vi "Strings and Values.vi"(8 "error in (no error)":errorcluster, 11 "NCDC Weather in":refnum<class "NCDC Weather.lvclass">) -> (0 "error out":errorcluster, 2 "Strings And Values []":T3, 3 "NCDC Weather out":refnum<class "NCDC Weather.lvclass">)   [LabVIEW 2020, in "NCDC Weather.lvclass"]
uses:
  NCDC Weather.lvclass
  <vilib>/Utility/miscctls.llb/LVComboBoxStrsAndValuesArrayTypeDef.ctl
  Location Result JSON.ctl
  Locations Results JSON.ctl
  NCDC Weather.lvclass/NCDC Weather.ctl
  <vilib>/httpClient/LabVIEWHTTPClient.lvlib
panel:
  out "Response (debug)":T1
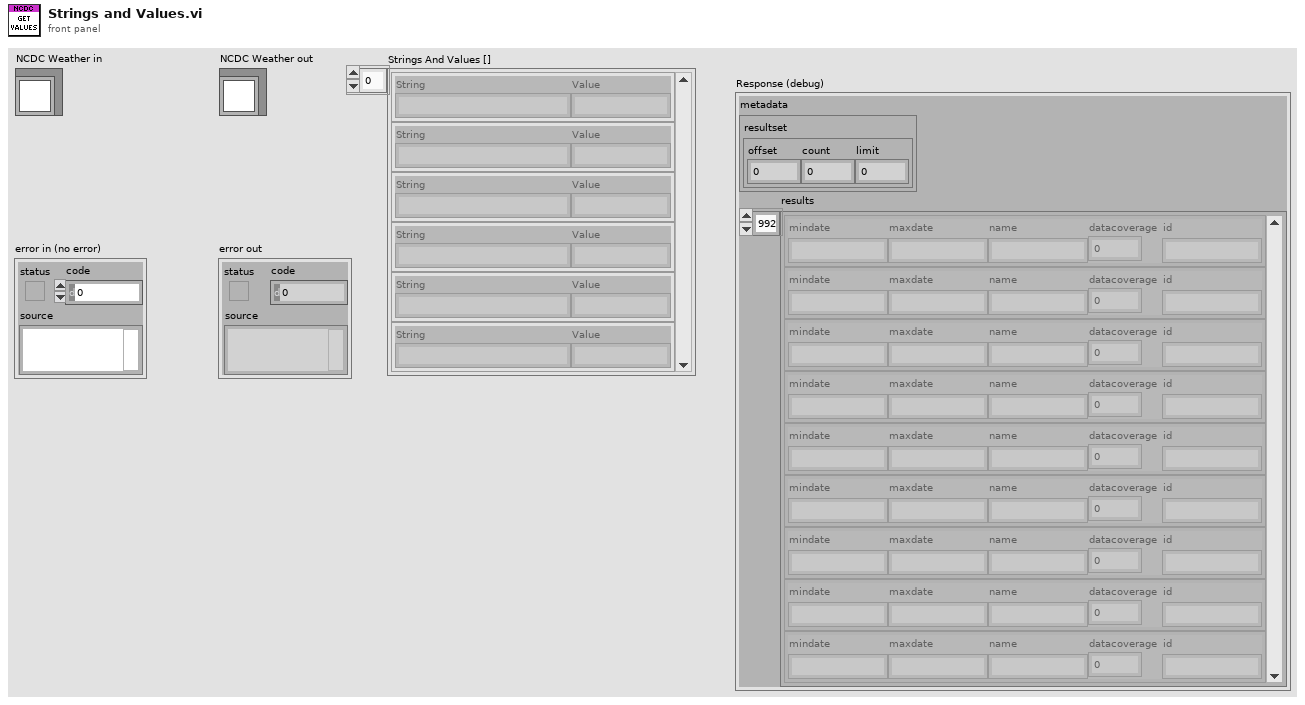
[diagram p1: front panel]
types:
  T1 = typedef "NCDC Weather.lvclass/Location Result JSON.ctl" = cluster{"metadata":cluster{"resultset":cluster{"offset":i32, "count":i32, "limit":i32}}, "results":T2[]}
  T2 = typedef "NCDC Weather.lvclass/Locations Results JSON.ctl" = cluster{"mindate":string, "maxdate":string, "name":string, "datacoverage":dbl, "id":string}
  T3 = typedef "LVComboBoxStrsAndValuesArrayTypeDef.ctl" = cluster{"String":string, "Value":string}[]
  T4 = typedef "LabVIEWHTTPClient.lvlib/ClientHandle.ctl" = refnum<k1>
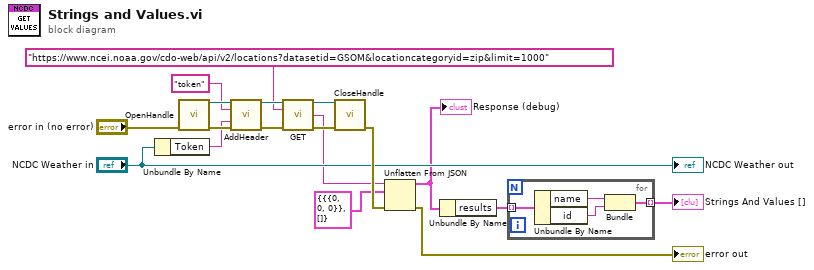
[diagram p0: block diagram]
diagram:
  n1 = Unbundle By Name("NCDC Weather in") -> ("Token"=w2:string)
  n2 = call <vilib>:"OpenHandle.vi"("error in (no error)"="error in (no error)") -> ("client handle out"=w16:T4, "error out"=w17:errorcluster)  [unwired: 13 in]
  n3 = call <vilib>:"AddHeader.vi"("client handle"=w16, "header"="token", "value"=w2, "error in (no error)"=w17) -> ("client handle out"=w14:T4, "error out"=w12:errorcluster)  [unwired: 10 in]
  n4 = call <vilib>:"GET.vi"("client handle"=w14, "url"="https://www.ncei.noaa.gov/cdo-web/api/v2/locations?datasetid=GSOM&locationcategoryid=zip&limit=1000", "error in (no error)"=w12) -> ("client handle out"=w11:T4, "body"=w7:string, "error out"=w10:errorcluster)  [unwired: 9 in, 1 out]
  n5 = call <vilib>:"CloseHandle.vi"("client handle"=w11, "error in (no error)"=w10) -> ("error out"=w18:errorcluster)  [unwired: 13 in]
  n6 = Unflatten From JSON(JSON string=w7, type and defaults=T1 {"metadata"={"resultset"={"offset"=0, "count"=0, "limit"=0}}, "results"=[]} ("Locations Result JSON"), error in (no error)=w18) -> (value=w6:T1, error out=→"error out":errorcluster)  [unwired: 4 in]
  "Response (debug)" <- w6
  n7 = Unbundle By Name(w6) -> ("results"=w5:T2[])
  n8 = for {
    tunnel: w5 -> [w22] mode=indexing
    tunnel: [w19] -> w4 mode=indexing
    n9 = Unbundle By Name(w22) -> ("name"=w21:string, "id"=w20:string)
    n10 = Bundle("name"=w21, "id"=w20) -> (w19:cluster{"name":string, "id":string})  [unwired: 1 in]
  }
  "Strings And Values []" <- w4
  "NCDC Weather out" <- "NCDC Weather in"
